vi "Teleop.vi"(10 "Match Info":T1={"Autonomous Elapsed Seconds"=0.0, "TeleOp Elapsed Seconds"=0.0, "Disabled Elapsed Seconds"=0.0, "Visited Autonomous"=FALSE, "Visited TeleOp"=FALSE, "Visited Disabled"=FALSE, "Autonomous Settings"={"Autonomous Style"=enum."Independent", "VI Refnum"=refnum}}, 11 "Call Context":T2) -> ()   [LabVIEW 2014]
doc: "This VI is called for each TeleOp packet received from the DS where the robot is not disabled. It is often used to read from the joysticks and update I/O or to update setpoints for timed control loops. It should complete and return within 20 milliseconds or it may miss DS packets."
uses:
  <vilib>/Rock Robotics/WPI/DriverStation/WPI_DriverStationDerivedRobotMode.ctl
  <vilib>/Rock Robotics/WPI/DriverStation/WPI_DriverStationMatch Info.ctl
  <vilib>/Rock Robotics/WPI/RobotDrive/WPI_RobotDriveGetSetRefNum.vi
  <vilib>/Rock Robotics/WPI/Joystick/WPI_JoystickGetSetRefNum.vi
  <vilib>/Rock Robotics/Network Tables/SD Write Boolean Array.vi
  <vilib>/Rock Robotics/Network Tables/SD Write Numeric Array.vi
  <vilib>/Rock Robotics/Network Tables/SD Read Boolean.vi
  <vilib>/Rock Robotics/Network Tables/SD Read Number.vi
  <vilib>/Rock Robotics/Network Tables/SD Write Number.vi
  <vilib>/Rock Robotics/WPI/RobotDrive/WPI_RobotDriveMecanumDrive_Cartesian.vi
  robotics/labview/nav6/roborio/labview/Nav6Library/Nav6.lvlib
panel:
  out "IsConnected":bool
  out "Byte Count":u32
  out "Update Count":i32
  out "Compass Heading":dbl
  out "Roll":dbl
  out "Pitch":dbl
  out "Sample Slider 0":dbl(slide) scale=0.0..5.0
  out "Sample Boolean 1":bool
  out "Sample Boolean 0":bool
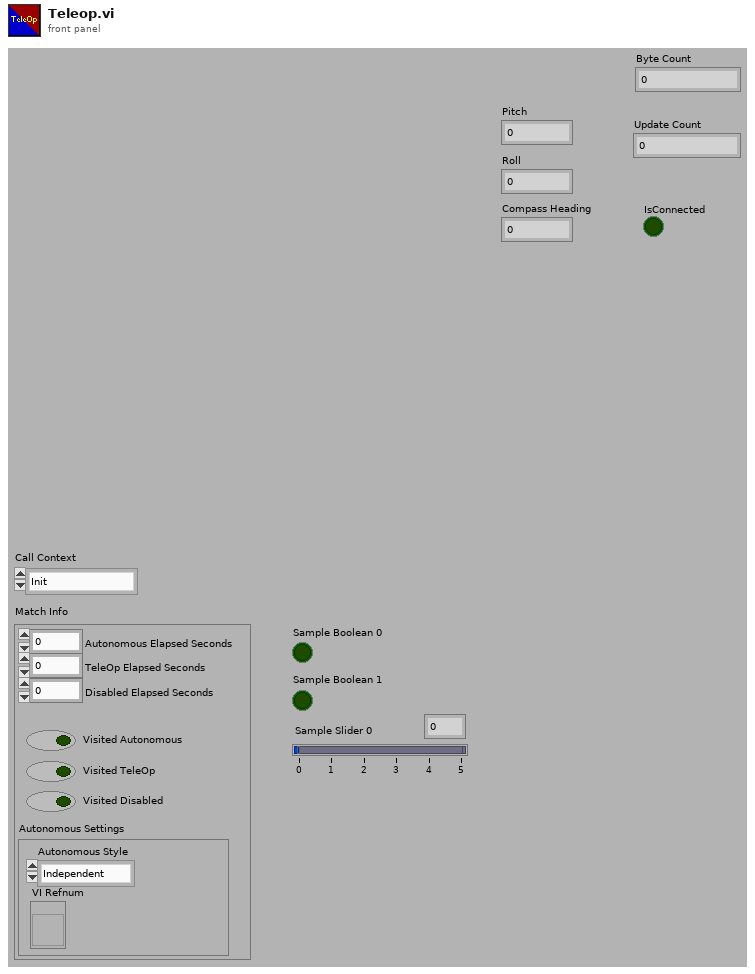
[diagram p1: front panel]
types:
  T1 = typedef "WPI_DriverStationMatch Info.ctl" = cluster{"Autonomous Elapsed Seconds":dbl, "TeleOp Elapsed Seconds":dbl, "Disabled Elapsed Seconds":dbl, "Visited Autonomous":bool, "Visited TeleOp":bool, "Visited Disabled":bool, "Autonomous Settings":cluster{"Autonomous Style":enum16{"Iterative", "Independent"}, "VI Refnum":refnum<vi>}}
  T2 = typedef "WPI_DriverStationDerivedRobotMode.ctl" = enum16{"Init", "Execute", "Stop"}
  T3 = typedef "WPI_RobotDriveDevRef.ctl" = cluster{"DevStatus":errorcluster, "Motors[]":T4[], "Square Inputs":bool, "Max Output":dbl}
  T4 = typedef "WPI_MotorControlDeviceRef.ctl" = cluster{"DeviceStatus":errorcluster, "Type":T5, "PWM":cluster{"Controller":T6, "PWM Channel":T7, "DeadBand":T8}, "CAN":cluster{"Device Number":u8, "Control Mode":T9, "Semaphore":T10, "Max Vout":dbl, "TalonSRX Control Mode":T11}, "Invert":bool, "TransformRef":T12, "InvTransformRef":T12}
  T5 = typedef "WPI_MotorControlType.ctl" = enum16{"PWM", "CAN", "CANTalonSRX"}
  T6 = typedef "FPGA_TypedefDigitalModule.ctl" = enum16{"Controller 1"}
  T7 = typedef "FPGA_DIOPWMChannel.ctl" = enum8{"PWM 0", "PWM 1", "PWM 2", "PWM 3", "PWM 4", "PWM 5", "PWM 6", "PWM 7", "PWM 8", "PWM 9", "PWM MXP 0", "PWM MXP 1", "PWM MXP 2", "PWM MXP 3", "PWM MXP 4", "PWM MXP 5", "PWM MXP 6", "PWM MXP 7", "PWM MXP 8", "PWM MXP 9", "Invalid"}
  T8 = typedef "WPI_PWMDeadband.ctl" = cluster{"Name":string, "maxPositivePwm":i32, "minPositivePwm":i32, "centerPwm":i32, "maxNegativePwm":i32, "minNegativePwm":i32, "angularRange":u16}
  T9 = typedef "WPI_CANJaguar_ControlMode.ctl" = enum8{"Percent VBus", "Current", "Speed", "Position", "Voltage"}
  T10 = typedef "Semaphore RefNum" = refnum<k1>
  T11 = typedef "WPI_CANTalonSRX_APIControlMode.ctl" = enum8{"Percent VBus", "Speed", "Position", "Slave", "Unchanged / Invalid"}
  T12 = typedef "WPI_PWMTransform_ConPane.ctl" = refnum<vi>
  T13 = typedef "WPI_JoystickDevRef.ctl" = cluster{"Device":T14}
  T14 = typedef "WPI_JoystickDeviceEnum.ctl" = enum16{"USB 0", "USB 1", "USB 2", "USB 3", "USB 4", "USB 5"}
  T15 = typedef "Nav6.lvlib/Nav6DevRef.ctl" = cluster{"SerialPortRef":T16, "UpdateRate":u8, "Error":errorcluster, "Nav6Mode":T17}
  T16 = typedef "WPI_SerialPortRef.ctl" = cluster{"DevStatus":errorcluster, "Serial Port Name":refnum<visa-resource-name>}
  T17 = typedef "Nav6.lvlib/Nav6Mode.ctl" = enum16{"YPR", "Gyro", "Quaternion"}
  T18 = typedef "WPI_AnalogChannelDevRef.ctl" = cluster{"DevStatus":errorcluster, "Controller":T19, "Analog Channel":T20}
  T19 = typedef "FPGA_TypedefAnalogModule.ctl" = enum16{"Controller 1"}
  T20 = typedef "FPGA_AIChannel.ctl" = enum8{"AI 0", "AI 1", "AI 2", "AI 3", "AI MXP 0", "AI MXP 1", "AI MXP 2", "AI MXP 3", "Invalid"}
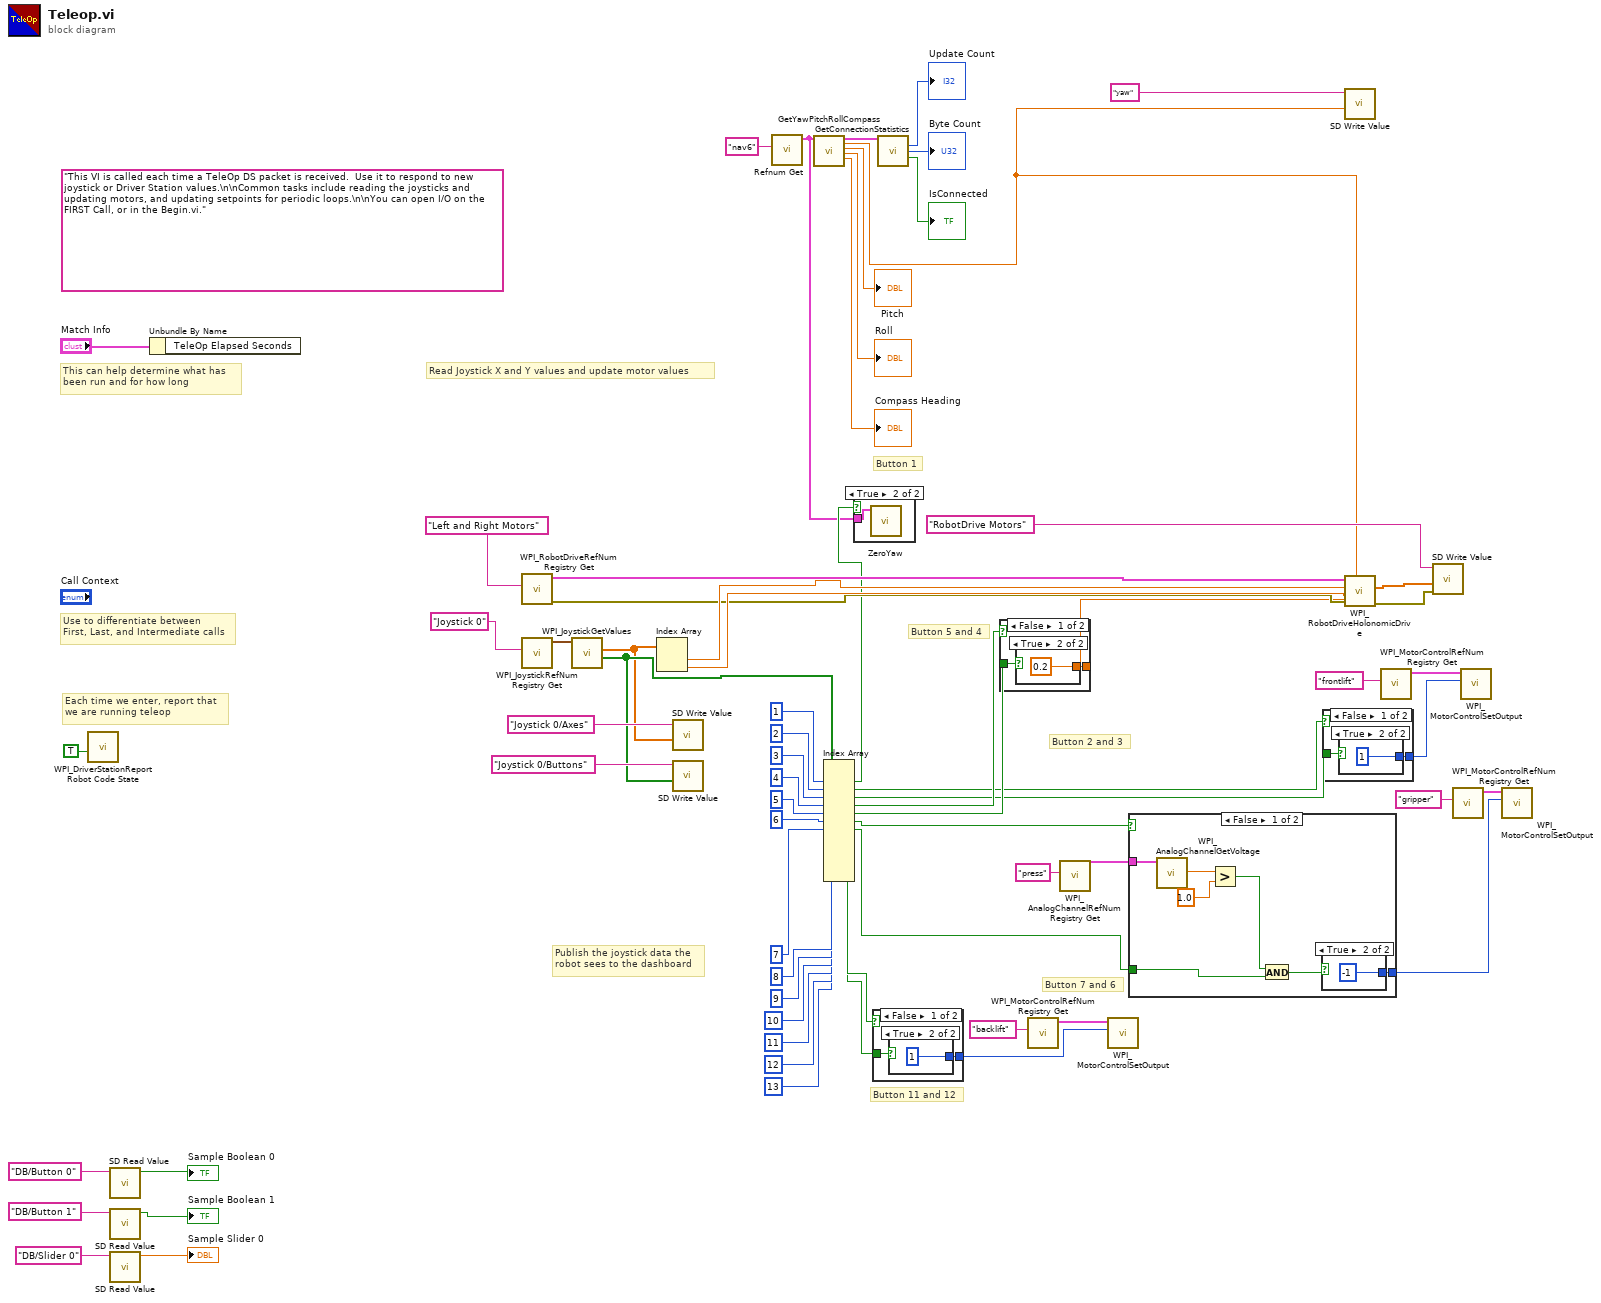
[diagram p0: block diagram]
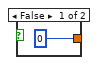
[diagram p3: hidden frame]
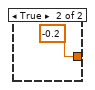
[diagram p4: hidden frame]
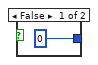
[diagram p5: hidden frame]
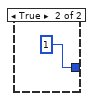
[diagram p6: hidden frame]
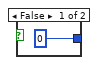
[diagram p7: hidden frame]
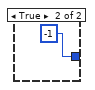
[diagram p8: hidden frame]
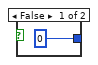
[diagram p9: hidden frame]
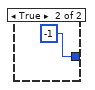
[diagram p10: hidden frame]
diagram:
  (unwired) "This VI is called each time a TeleOp DS packet is received.  Use it to respond to new joystick or Driver Station values.\n\nCommon tasks include reading the joysticks and updating motors, and updating setpoints for periodic loops.\n\nYou can open I/O on the FIRST Call, or in the Begin.vi."
  # "Button 11 and 12"
  # "Button 7 and 6"
  # "Button 2 and 3"
  # "Button 5 and 4"
  # "Button 1"
  # "Publish the joystick data the\nrobot sees to the dashboard"
  # "Each time we enter, report that\nwe are running teleop"
  # "Use to differentiate between\nFirst, Last, and Intermediate calls"
  # "This can help determine what has\nbeen run and for how long"
  # "Read Joystick X and Y values and update motor values"
  n1 = call <vilib>:"WPI_DriverStationReport Robot Code State.vi"("TeleOp"=TRUE ("Autonomous")) -> ()  [unwired: 10 in, 1 out]
  n2 = call-poly <vilib>:"SD Read Value.vi"("Name"="DB/Button 0" ("refnum name")) -> ("Boolean"=→"Sample Boolean 0":bool)  [unwired: 8 in, 2 out]
  n3 = call-poly <vilib>:"SD Read Value.vi"("Name"="DB/Button 1" ("refnum name")) -> ("Boolean"=→"Sample Boolean 1":bool)  [unwired: 8 in, 2 out]
  n4 = call-poly <vilib>:"SD Read Value.vi"("Name"="DB/Slider 0" ("refnum name")) -> ("Numeric"=→"Sample Slider 0":dbl)  [unwired: 8 in, 2 out]
  n5 = Unbundle By Name("Match Info") -> ()  [unwired: 1 out]
  n6 = call <vilib>:"WPI_RobotDriveRefNum Registry Get.vi"("refnum name"="Left and Right Motors") -> ("error out"=w48:errorcluster, "RobotDriveDevRef"=w51:T3)  [unwired: 1 in, 8 out]
  n7 = call <vilib>:"WPI_JoystickRefNum Registry Get.vi"("refnum name"="Joystick 0") -> ("JoystickDevRef"=w64:T13)  [unwired: 1 in, 9 out]
  n8 = call <vilib>:"WPI_JoystickGetValues.vi"("JoystickDevRef"=w64) -> ("Buttons"=w14:bool[], "Axes"=w13:dbl[])  [unwired: 6 in, 3 out]
  n9 = Index Array(array=w13) -> (element #1=w50:dbl, element #2=w49:dbl)  [unwired: 2 in]
  n10 = call-poly <vilib>:"SD Write Value.vi"("Numeric Array"=w13, "Name"="Joystick 0/Axes") -> ()  [unwired: 8 in, 2 out]
  n11 = call-poly <vilib>:"SD Write Value.vi"("Boolean Array"=w14, "Name"="Joystick 0/Buttons") -> ()  [unwired: 8 in, 2 out]
  n12 = call "Refnum Get.vi"("refnum name"="nav6") -> ("Nav6DevRef"=w11:T15)  [unwired: 9 in, 1 out]
  n13 = call "GetYawPitchRollCompass.vi"("Nav6DevRef"=w11) -> ("Nav6DevRef Out"=w39:T15, "Yaw"=w34:dbl, "Pitch"=→"Pitch":dbl, "Roll"=→"Roll":dbl, "Compass Heading"=→"Compass Heading":dbl)  [unwired: 12 in, 2 out]
  n14 = Index Array(array=w14, index #1=1 ("index"), index #2=2 ("index"), index #3=3 ("index"), index #4=4 ("index"), index #5=5 ("index"), index #6=6 ("index"), index #7=7 ("index"), index #8=8 ("index"), index #9=9 ("index"), index #10=10 ("index"), index #11=11 ("index"), index #12=12 ("index"), index #13=13 ("index")) -> (element #1=w12:bool, element #2=w8:bool, element #3=w7:bool, element #4=w10:bool, element #5=w9:bool, element #6=w6:bool, element #7=w5:bool, element #11=w4:bool, element #12=w3:bool)  [unwired: 4 out]
  n15 = case shown="True" w12 {
    tunnel: w11 -> [_ w68]
    frame False {
    }
    frame True {
      n16 = call "ZeroYaw.vi"("Nav6DevRef"=w68) -> ()  [unwired: 9 in, 2 out]
    }
  }
  n17 = case shown="False" w4 {
    tunnel: [w70 -1] -> w31
    tunnel: w3 -> [w69 _]
    frame False {
      n18 = case shown="True" w69 {
        tunnel: [0 1] -> w70
        frame False {
        }
        frame True {
        }
      }
    }
    frame True {
    }
  }
  n19 = call "GetConnectionStatistics.vi"("Nav6DevRef"=w39) -> ("Update Count"=→"Update Count":i32, "Byte Count"=→"Byte Count":u32, "IsConnected"=→"IsConnected":bool)  [unwired: 10 in, 2 out]
  n20 = case shown="False" w10 {
    tunnel: [w75 -0.2] -> w28
    tunnel: w9 -> [w74 _]
    frame False {
      n21 = case shown="True" w74 {
        tunnel: [0 0.2] -> w75
        frame False {
        }
        frame True {
        }
      }
    }
    frame True {
    }
  }
  n22 = call <vilib>:"WPI_MotorControlRefNum Registry Get.vi"("refnum name"="backlift") -> ("MotorControlDevRef"=w32:T4)  [unwired: 9 in, 1 out]
  n23 = call <vilib>:"WPI_AnalogChannelRefNum Registry Get.vi"("refnum name"="press") -> ("AIDeviceRef"=w1:T18)  [unwired: 9 in, 1 out]
  n24 = call <vilib>:"WPI_MotorControlSetOutput.vi"("Output"=w31, "MotorControlDevRef"=w32) -> ()  [unwired: 7 in, 3 out]
  n25 = case shown="False" w6 {
    tunnel: [w85 1] -> w29
    tunnel: w5 -> [w79 _]
    tunnel: w1 -> [w84 _]
    frame False {
      n26 = call <vilib>:"WPI_AnalogChannelGetVoltage.vi"("AIDeviceRef"=w84) -> ("Voltage"=w83:dbl)  [unwired: 8 in, 2 out]
      n27 = Greater?(x=w83, y=1.0) -> (0:w80:bool)
      n28 = And(x=w80, y=w79) -> (x .and. y?=w81:bool)
      n29 = case shown="True" w81 {
        tunnel: [0 -1] -> w85
        frame False {
        }
        frame True {
        }
      }
    }
    frame True {
    }
  }
  n30 = case shown="False" w8 {
    tunnel: [w90 -1] -> w30
    tunnel: w7 -> [w89 _]
    frame False {
      n31 = case shown="True" w89 {
        tunnel: [0 1] -> w90
        frame False {
        }
        frame True {
        }
      }
    }
    frame True {
    }
  }
  n32 = call-poly <vilib>:"SD Write Value.vi"("Numeric"=w34, "Name"="yaw" ("refnum name")) -> ()  [unwired: 8 in, 2 out]
  n33 = call-poly <vilib>:"WPI_RobotDriveHolonomicDrive.vi"("Rotation"=w28, "Gyro Angle"=w34, "error in (no error)"=w48, "Y"=w49, "X"=w50, "RobotDriveDevRef"=w51) -> ("error out"=w53:errorcluster, "Motor Values"=w52:dbl[])  [unwired: 3 in, 1 out]
  n34 = call <vilib>:"WPI_MotorControlRefNum Registry Get.vi"("refnum name"="frontlift") -> ("MotorControlDevRef"=w46:T4)  [unwired: 9 in, 1 out]
  n35 = call-poly <vilib>:"SD Write Value.vi"("error in"=w53, "Numeric Array"=w52, "Name"="RobotDrive Motors") -> ()  [unwired: 7 in, 2 out]
  n36 = call <vilib>:"WPI_MotorControlRefNum Registry Get.vi"("refnum name"="gripper") -> ("MotorControlDevRef"=w45:T4)  [unwired: 9 in, 1 out]
  n37 = call <vilib>:"WPI_MotorControlSetOutput.vi"("Output"=w30, "MotorControlDevRef"=w46) -> ()  [unwired: 7 in, 3 out]
  n38 = call <vilib>:"WPI_MotorControlSetOutput.vi"("Output"=w29, "MotorControlDevRef"=w45) -> ()  [unwired: 7 in, 3 out]
